vi "Actor-Caller.vi"(5 "Initialize-Error Passback":refnum<notifier>, 7 "Events Passback":refnum<notifier>, 9 "Stopped Event":refnum<user-event>, 10 "Launch":refnum<notifier>, 11 "Actor in":refnum<class "Actor.lvclass">) -> ()   [LabVIEW 2018, in "Actor.lvlib" / "Actor-Interface.lvclass"]
uses:
  Actor-Interface.lvclass
  Actor.lvclass
  Events.ctl
  Stop.ctl
  Launched.ctl
  Stopped.ctl
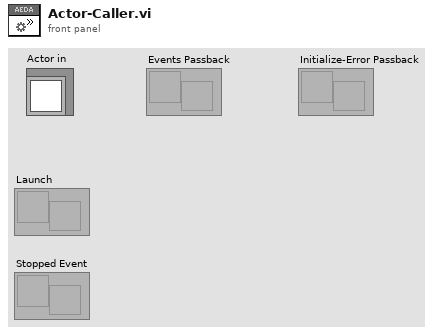
[diagram p1: front panel]
types:
  T1 = typedef "Actor.lvlib/Actor-Interface.lvclass/Stopped.ctl" = cluster{"Actor":refnum<class "Actor.lvclass">, "Final Error":errorcluster}
  T2 = typedef "Actor.lvlib/Actor-Interface.lvclass/Events.ctl" = cluster{"Stop":refnum<user-event>, "Launched":refnum<user-event>}
  T3 = typedef "Actor.lvlib/Actor-Interface.lvclass/Event-Registrations.ctl" = cluster{"Stop":refnum<event-registration>}
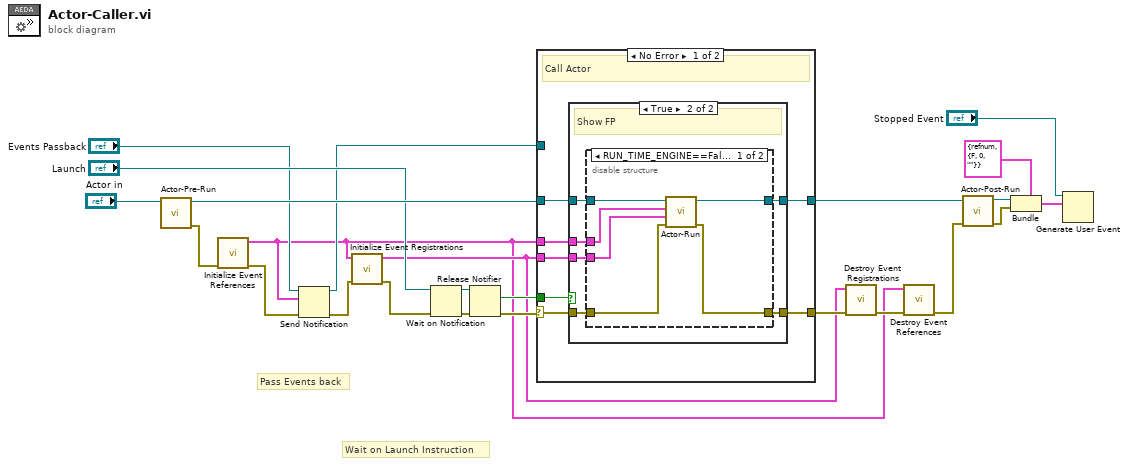
[diagram p0: block diagram]
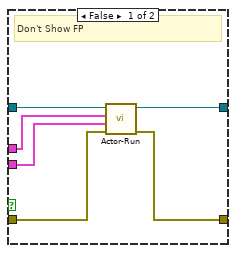
[diagram p2: hidden frame]
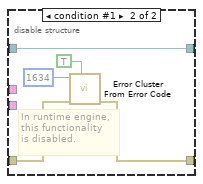
[diagram p3: hidden frame]
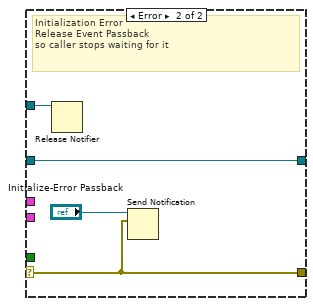
[diagram p4: hidden frame]
diagram:
  # "Wait on Launch Instruction"
  # "Pass Events back"
  n1 = call-dynamic "Actor-Pre-Run.vi"("Actor in"="Actor in") -> ("error out"=w6:errorcluster, "Actor out"=w24:refnum<class "Actor.lvclass">)  [unwired: 9 in]
  n2 = call "Initialize Event References.vi"("error in (no error)"=w6) -> ("error out"=w5:errorcluster, "Actor-Events"=w1:T2)  [unwired: 9 in]
  n3 = Send Notification(notification=w1, notifier="Events Passback", error in (no error)=w5) -> (notifier out=w7:refnum<notifier>, error out=w4:errorcluster)
  n4 = call "Initialize Event Registrations.vi"("error in (no error)"=w4, "Actor-Events"=w1) -> ("error out"=w3:errorcluster, "Actor-Event-Registrations"=w2:T3)  [unwired: 8 in]
  n5 = Wait on Notification(notifier="Launch", error in (no error)=w3) -> (notifier out=w21:refnum<notifier>, error out=w20:errorcluster)  [unwired: 2 in, 2 out]
  n6 = Release Notifier(notifier=w21, error in (no error)=w20) -> (last notification=w18:bool, error out=w19:errorcluster)  [unwired: 1 in, 1 out]
  n7 = case shown="No Error" w19 {
    selector: w19 -> [w27 w57]
    tunnel: w24 -> [w31 w58]
    tunnel: w7 -> [_ w56]
    tunnel: [w30 w57] -> w16
    tunnel: [w29 w58] -> w23
    tunnel: w18 -> [w28 _]
    tunnel: w2 -> [w25 _]
    tunnel: w1 -> [w26 _]
    frame No Error {
      # "Call Actor"
      n8 = case shown="True" w28 {
        tunnel: w31 -> [w37 w42]
        tunnel: [w36 w40] -> w30
        tunnel: [w35 w41] -> w29
        tunnel: w27 -> [w34 w43]
        tunnel: w26 -> [w33 w39]
        tunnel: w25 -> [w32 w38]
        frame False {
          # "Don't Show FP"
          n9 = call-dynamic "Actor-Run.vi"("error in"=w34, "Actor-Event-Registrations"=w32, "Actor-Events"=w33, "Actor in"=w37) -> ("error out"=w36:errorcluster, "Actor out"=w35:refnum<class "Actor.lvclass">)  [unwired: 6 in]
        }
        frame True {
          # "Show FP"
          n10 = disable-structure shown="RUN_TIME_ENGINE==False" {
            disable-tunnel: [w47 w53] -> w40
            disable-tunnel: [w46 w54] -> w41
            disable-tunnel: w42 -> [w49 w54]
            disable-tunnel: w43 -> [w48 w52]
            disable-tunnel: w39 -> [w45 _]
            disable-tunnel: w38 -> [w44 _]
            frame condition #0 (active) {
              n11 = call-dynamic "Actor-Run.vi"("error in"=w48, "Actor-Event-Registrations"=w44, "Actor-Events"=w45, "Actor in"=w49) -> ("error out"=w47:errorcluster, "Actor out"=w46:refnum<class "Actor.lvclass">)  [unwired: 6 in]
            }
            frame condition #1 {
              # "In runtime engine,\nthis functionality\nis disabled."
              n12 = call <vilib>:"Error Cluster From Error Code.vi"("show call chain? (False)"=TRUE, "error in (no error)"=w52, "error code (0)"=1634) -> ("error out"=w53:errorcluster)  [unwired: 6 in]
            }
          }
        }
      }
    }
    frame Error {
      # "Initialization Error\nRelease Event Passback\nso caller stops waiting for it"
      n13 = Release Notifier(notifier=w56) -> ()  [unwired: 2 in, 3 out]
      n14 = Send Notification(notification=w57, notifier="Initialize-Error Passback") -> ()  [unwired: 1 in, 2 out]
    }
  }
  n15 = call "Destroy Event Registrations.vi"("error in (no error)"=w16, "Actor-Event-Registrations"=w2) -> ("error out"=w15:errorcluster)  [unwired: 9 in]
  n16 = call "Destroy Event References.vi"("error in (no error)"=w15, "Actor-Events"=w1) -> ("error out"=w17:errorcluster)  [unwired: 9 in]
  n17 = call-dynamic "Actor-Post-Run.vi"("error in"=w17, "Actor in"=w23) -> ("error out"=w11:errorcluster, "Actor out"=w12:refnum<class "Actor.lvclass">)  [unwired: 8 in]
  n18 = Bundle(cluster=T1 {"Actor"=refnum, "Final Error"={"status"=FALSE, "code"=0, "source"=""}} ("event data"), "Actor"=w12, "Final Error"=w11) -> (w13:T1)
  n19 = Generate User Event(user event="Stopped Event", event data cluster=w13) -> ()  [unwired: 2 in, 2 out]
